vi "Reset Q0.vi"(8 "error in (no error)":errorcluster, 11 "Scope5761 in":refnum<class "Scope5782_six_channel.lvclass">) -> (0 "error out":errorcluster, 3 "Scope5761out":refnum<class "Scope5782_six_channel.lvclass">)   [LabVIEW 2018, in "Scope5782_six_channel.lvclass"]
uses:
  Scope5782_six_channel.lvclass
  Scope5782_six_channel.lvclass/Scope5782_six_channel.ctl
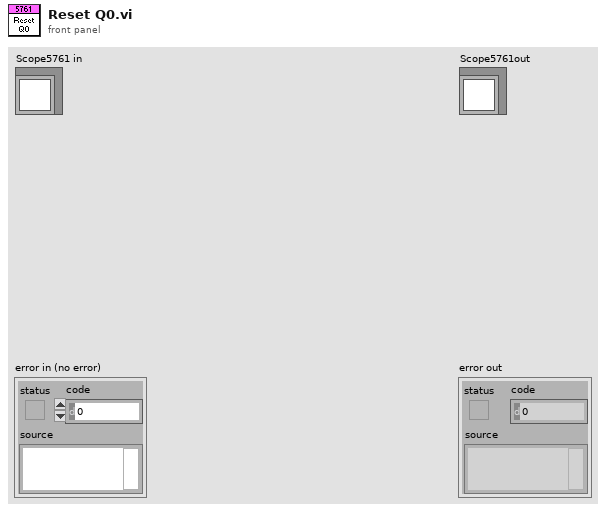
[diagram p1: front panel]
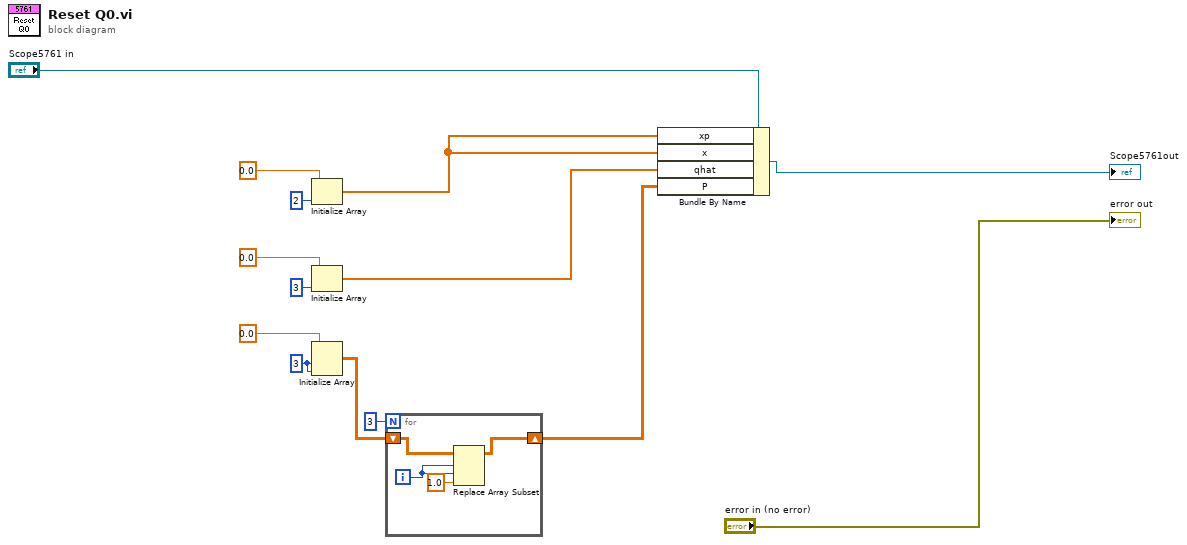
[diagram p0: block diagram]
diagram:
  w6 = 3 ("dimension size")
  n1 = Initialize Array(0.0 ("element"), 2 ("dimension size")) -> (w11:dbl[])
  n2 = Initialize Array(0.0 ("element"), 3 ("dimension size")) -> (w8:dbl[])
  n3 = Initialize Array(0.0 ("element"), w6, w6) -> (w3:dbl[][])
  n4 = for {
    N: 3 -> [_]
    shift-right: [w17] -> w2
    shift-left: w3 -> [w18]
    i -> [w16]
    n5 = Replace Array Subset(array=w18, new element=1.0 ("new element/subarray"), index (row)=w16, index (col)=w16) -> (w17:dbl[][])
  }
  n6 = Bundle By Name(cluster="Scope5761 in", "xp"=w11, "x"=w11, "qhat"=w8, "P"=w2) -> (→"Scope5761out":refnum<class "Scope5782_six_channel.lvclass">)
  "error out" <- "error in (no error)"
